vi "D999_Alone.vi"(8 "error in (no error)":errorcluster) -> (0 "error out":errorcluster)   [LabVIEW 2018]
uses:
  RT/PublicSubVI/Ctl/_ctl_RT_D999_Param.ctl
  <resource>/objmgr/ni.var.rc
  <vilib>/Utility/miscctls.llb/LVBoundsTypeDef.ctl
panel:
  in  "D999_list":i32(listbox)=-1
  in  "Load":bool
  in  "Save":bool
  in  "Label":string[](array[string])=["", "", "", "", "", "", "", "", "", "", "", ""]
  in  "AI":string[](array[string])=["AI 0", "AI 1", "AI 2", "AI 3", "AI 4", "AI 5", "AI 6", "AI 7", "AI 8", "AI 9", "AI 10", "AI 11"]
  in  "Multiply":dbl[](array[numeric])=[1.0, 1.0, 1.0, 1.0, 1.0, 1.0, 1.0, 1.0, 1.0, 1.0, 1.0, 1.0]
  in  "Add":dbl[](array[numeric])=[0.0, 0.0, 0.0, 0.0, 0.0, 0.0, 0.0, 0.0, 0.0, 0.0, 0.0, 0.0]
  in  "Enable":bool
  in  "AO":string[](array[string])=["AO 0", "AO 1", "AO 2", "AO 3", "AO 4", "AO 5", "AO 6", "AO 7", "AO 8"]
  in  "WriteValue":i16[](array[numeric])=[0, 0, 0, 0, 0, 0, 0, 0, 0] min=-4095 max=4095
  in  "WriteColor":u32[](array[colorbox])=[16777224, 16777224, 16777224, 16777224, 16777224, 16777224, 16777224, 16777224, 16777224]
  in  "Scale":u16=1 min=1
  in  "CEM(AO1)":bool
  in  "DYNODE(AO 0)":bool
  in  "ESPY(AO2)":bool
  in  "LENS(AO 3 : AO 8)":bool
  in  "Description":string="LENS : OFF; ESPY : OFF; DYNODE : OFF; CEN : OFF; "
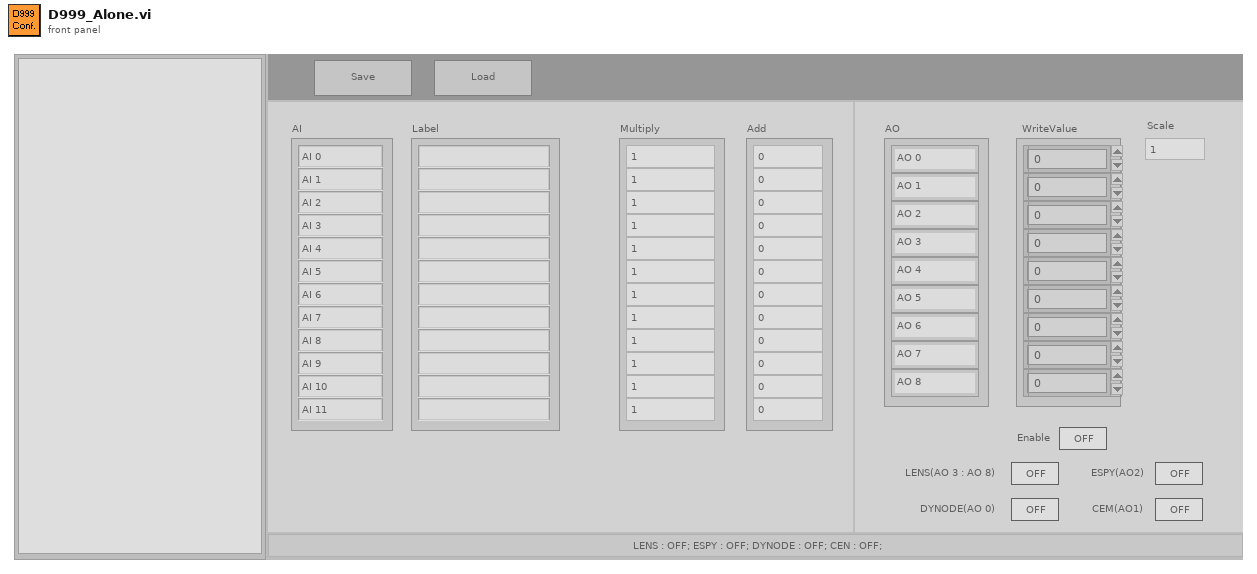
[diagram p1: front panel]
types:
  T1 = cluster{"Enable":refnum<vi>, "Label":refnum<vi>, "Multiply":refnum<vi>, "Add":refnum<vi>, "WriteColor":refnum<vi>, "WriteValue":refnum<vi>, "Description":refnum<vi>, "switch array":refnum<vi>[]}
  T2 = enum8{"Enabled", "Disabled", "Disabled and Grayed Out"}
  T3 = enum32{"Invalid", "Default", "Floating", "Floating/Auto-Hide", "Modal"}
  T4 = typedef "LVBoundsTypeDef.ctl" = cluster{"Width":u32, "Height":u32}
  T5 = cluster{"Label":string, "MultiValue":dbl, "AddValue":dbl}
  T6 = typedef "_ctl_RT_D999_Param.ctl" = cluster{"Enable":bool, "AI":cluster{"Label":string, "MultiValue":dbl, "AddValue":dbl}[], "AO":i16[], "Switch":bool[]}
  T7 = cluster{"Label":string[], "Multiply":dbl[], "Add":dbl[], "WriteValue":i16[], "switch":u32}
  T8 = typedef "eventvkey.ctl" = enum16{"ASCII", "Enter", "Return", "Shift", "Ctrl", "Alt", "Cmd", "Opt", "Caps", "NumLock", "Clear", "Break", "Up", "Down", "Left", "Right", "Insert", "Delete", "Home", "End", "PageUp", "PageDown", "Escape", "Help", "Pause", "ScrollLock", "F1", "F2", "F3", "F4", "F5", "F6", "F7", "F8", "F9", "F10", "F11", "F12", "F13", "F14", "F15", "F16", "F17", "F18", "F19", "F20", "F21", "F22", "F23", "F24", "Play", "VolumeUp", "VolumeDown", "Mute", "Two Byte Char"}
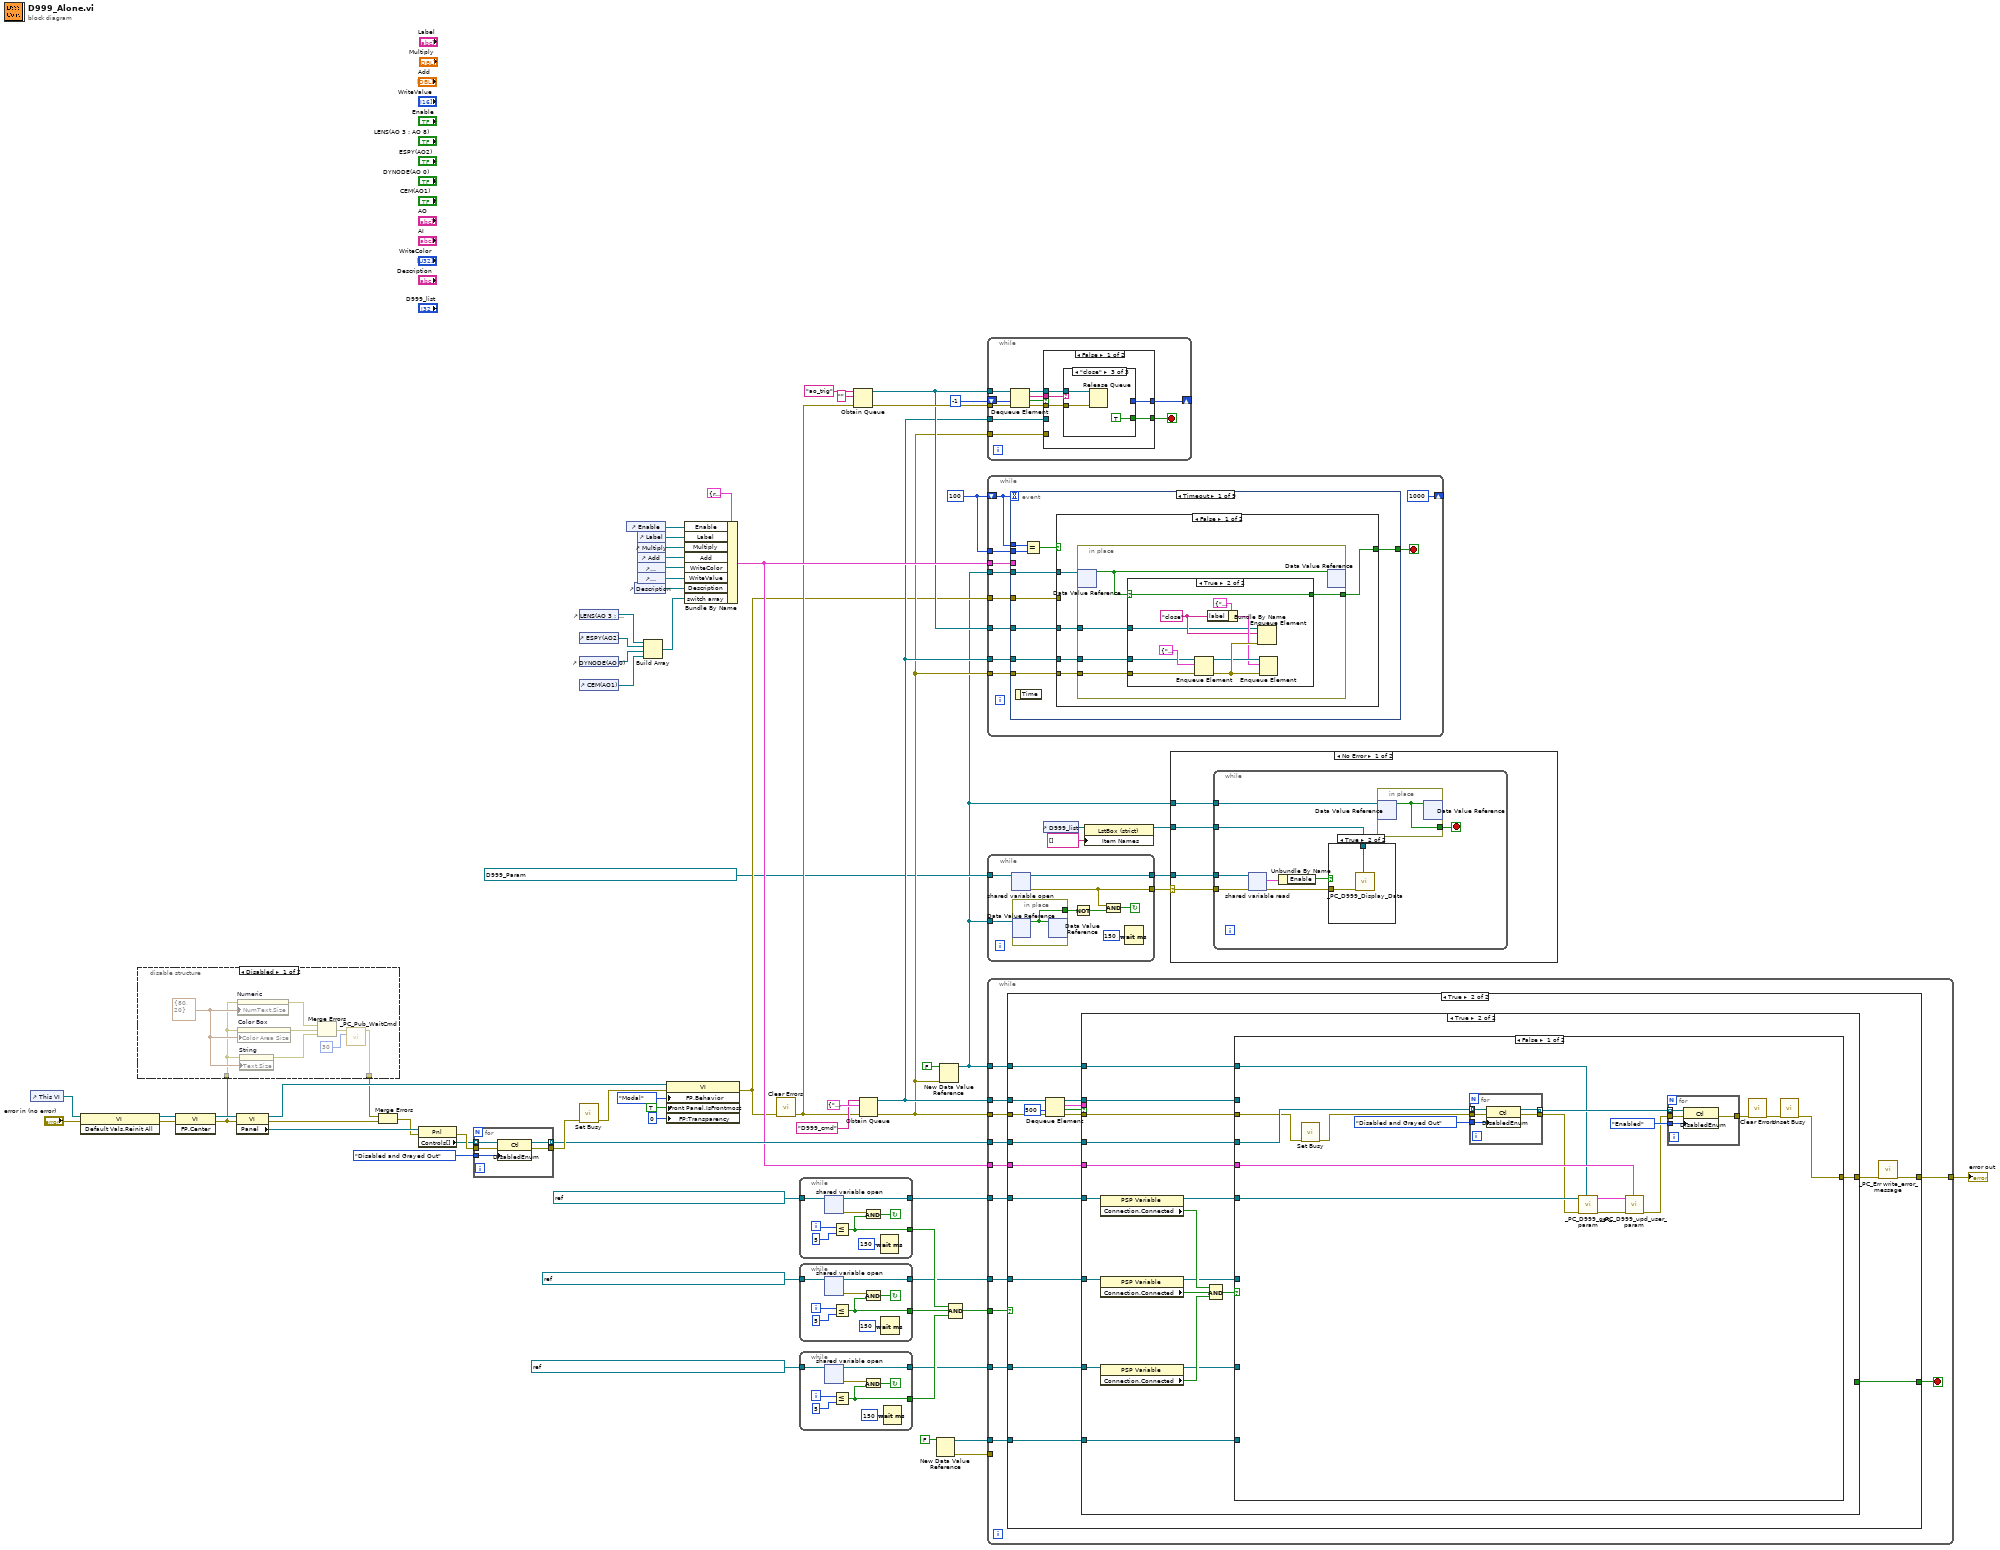
[diagram p0: block diagram]
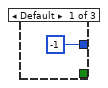
[diagram p5: hidden frame]
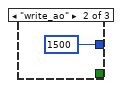
[diagram p6: hidden frame]
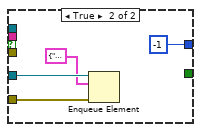
[diagram p7: hidden frame]
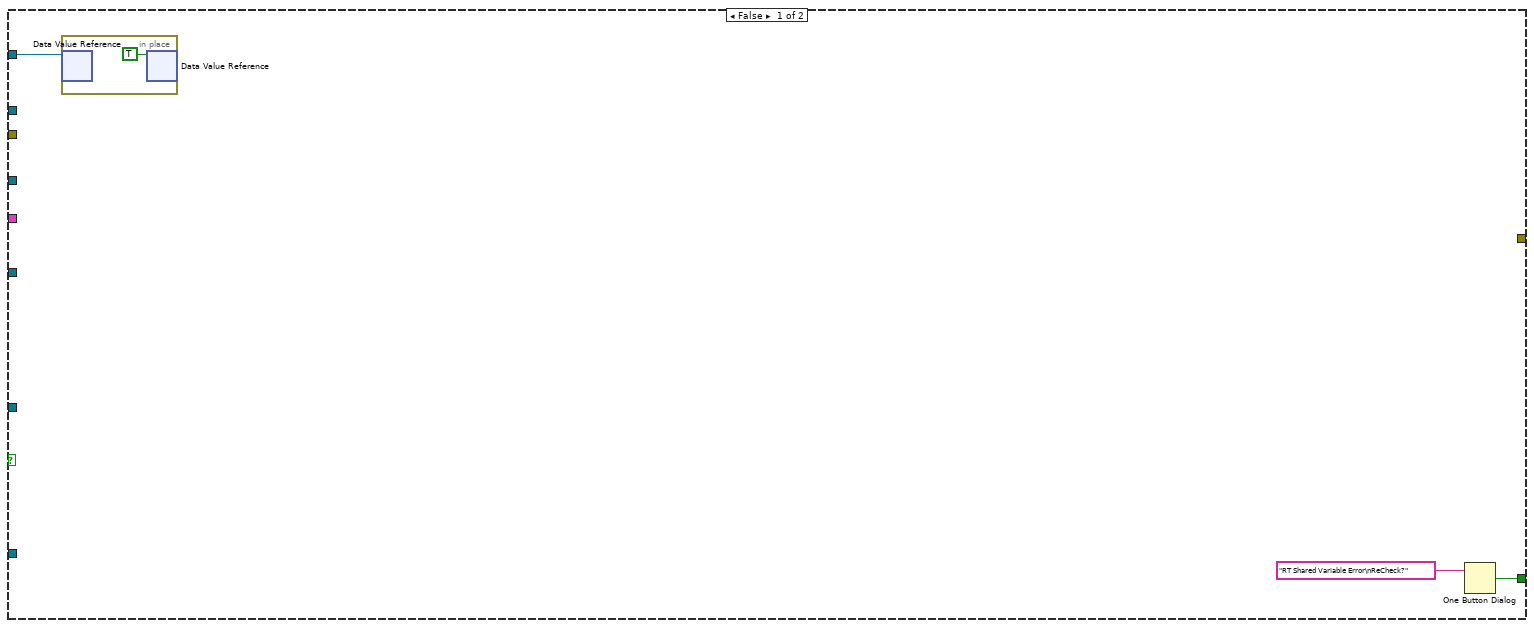
[diagram p8: hidden frame]
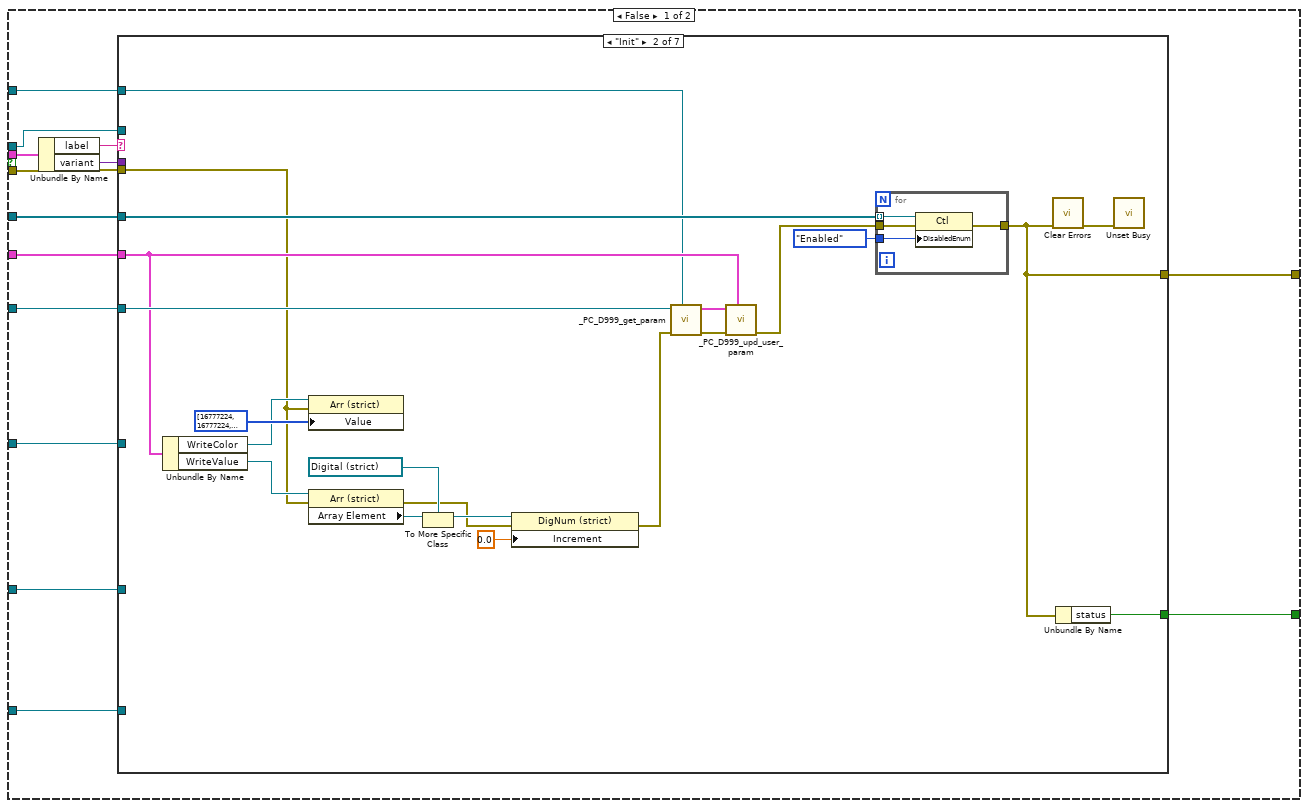
[diagram p9: hidden frame]
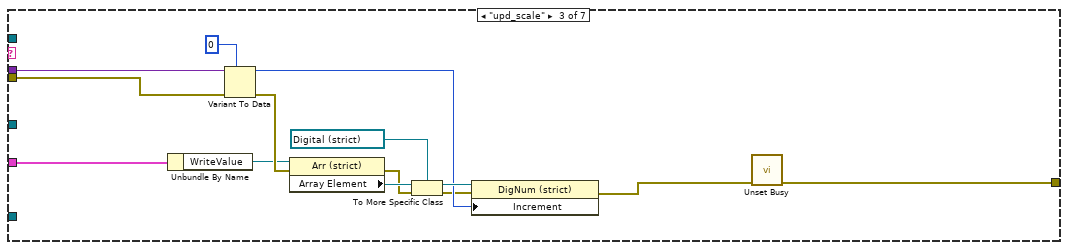
[diagram p11: hidden frame]
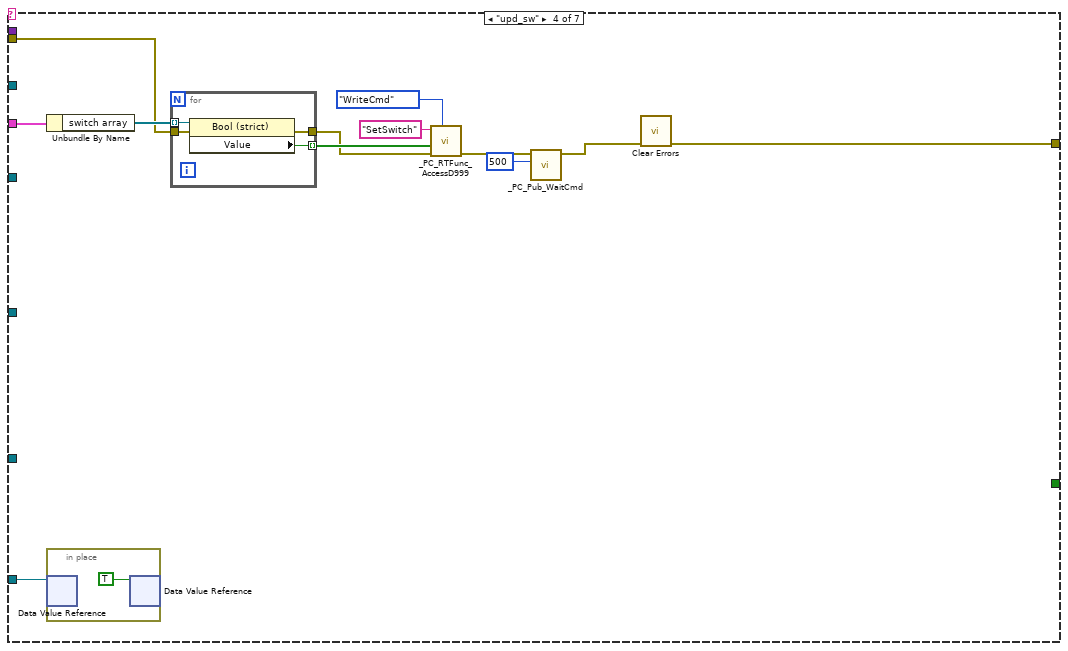
[diagram p12: hidden frame]
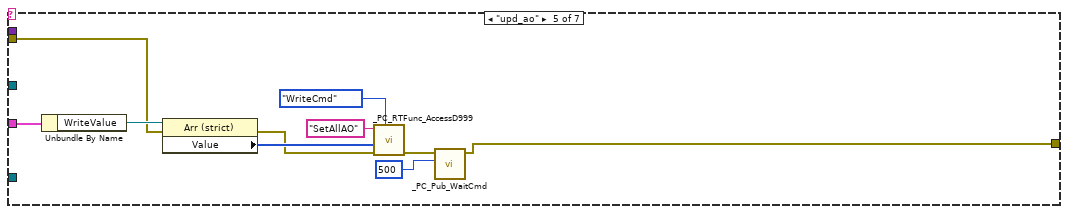
[diagram p13: hidden frame]
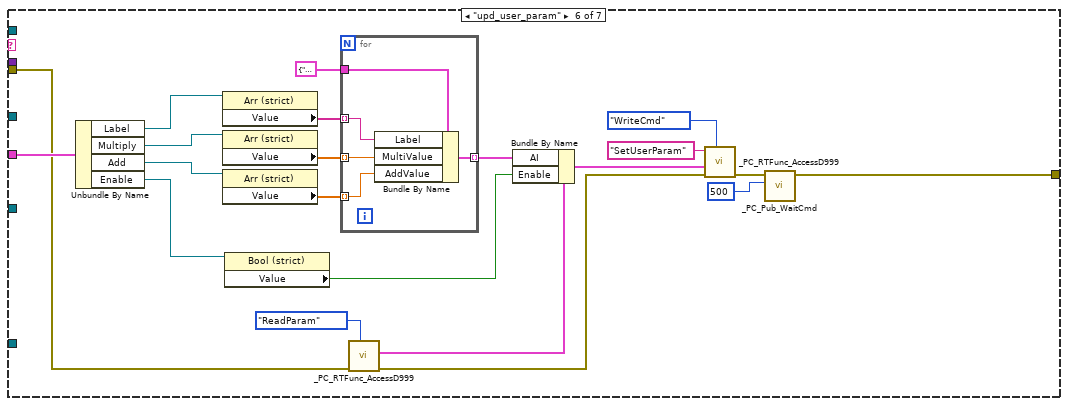
[diagram p14: hidden frame]
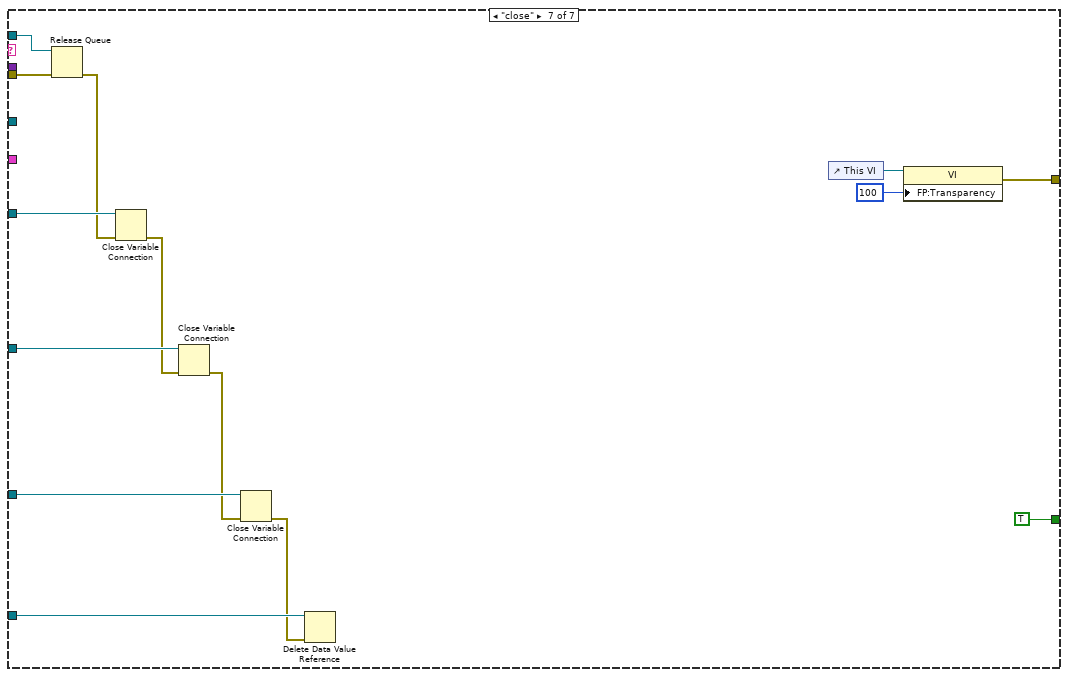
[diagram p15: hidden frame]
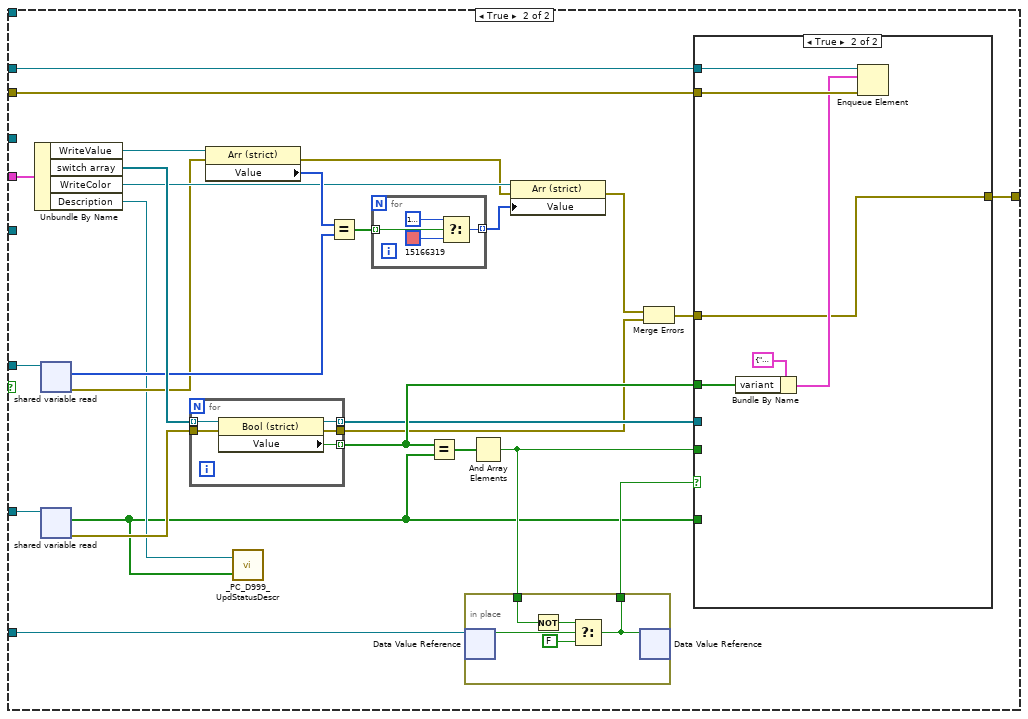
[diagram p16: hidden frame]
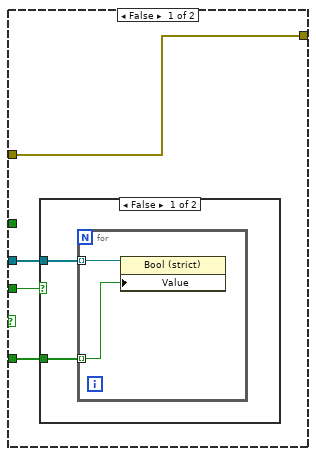
[diagram p17: hidden frame]
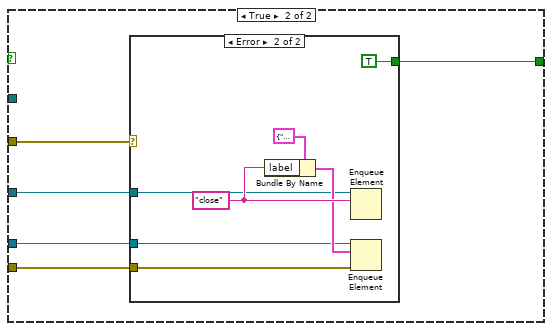
[diagram p20: hidden frame]
diagram:
  w4 = 100
  n1 = control-ref of="This VI"() -> (w65:refnum<vi>)
  n2 = invoke class="VI" method="Default Vals.Reinit All"(reference=w65, error in="error in (no error)") -> (reference out=w66:refnum<vi>, error out=w63:errorcluster)  [unwired: 1 in, 1 out]
  n3 = invoke class="VI" method="FP.Center"(reference=w66, error in=w63) -> (reference out=w58:refnum<vi>, error out=w15:errorcluster)  [unwired: 1 in, 1 out]
  n4 = disable-structure shown="Disabled" {
    disable-tunnel: w15 -> [w70 w77]
    disable-tunnel: [w69 w77] -> w12
    frame Disabled {
      w76 = T4 {"Width"=80, "Height"=20} ("Numeric Text.Size")
      n5 = property on="Numeric" class="DigNum (strict)"(error in=w70, "NumText.Size"=w76) -> (error out=w75:errorcluster)  [unwired: 1 in, 1 out]
      n6 = property on="Color Box" class="ColBox"(error in=w70, "Color Area Size"=w76) -> (error out=w74:errorcluster)  [unwired: 1 in, 1 out]
      n7 = property on="String" class="Str"(error in=w70, "Text.Size"=w76) -> (error out=w73:errorcluster)  [unwired: 1 in, 1 out]
      n8 = Merge Errors(w75, w74, w73) -> (w71:errorcluster)
      n9 = call "_PC_Pub_WaitCmd.vi"("milliseconds to wait"=u32 30, "error in (no error)"=w71) -> ("error out"=w69:errorcluster)  [unwired: 9 in]
    }
    frame Enabled {
    }
  }
  n10 = property class="VI"(reference=w58, error in=w15) -> (reference out=w57:refnum<vi>, error out=w13:errorcluster, "Panel"=w64:refnum<vi>)
  n11 = Merge Errors(w12, w13) -> (w11:errorcluster)
  n12 = property class="Pnl"(reference=w64, error in=w11) -> (error out=w61:errorcluster, "Controls[]"=w60:refnum<vi>[])  [unwired: 1 out]
  n13 = for {
    tunnel: w60 -> [w82] mode=indexing
    tunnel: T2."Disabled and Grayed Out" ("Disabled") -> [w81]
    tunnel: [w80] -> w29 mode=indexing
    tunnel: [w79] -> w56
    tunnel: w61 -> [w78]
    n14 = property class="Ctl"(reference=w82, error in=w78, "DisabledEnum"=w81) -> (reference out=w80:refnum<vi>, error out=w79:errorcluster)
  }
  n15 = control-ref of="LENS(AO 3 : AO 8)"() -> (w40:refnum<vi>)
  n16 = control-ref of="ESPY(AO2)"() -> (w41:refnum<vi>)
  n17 = control-ref of="DYNODE(AO 0)"() -> (w42:refnum<vi>)
  n18 = control-ref of="CEM(AO1)"() -> (w43:refnum<vi>)
  n19 = call <vilib>:"Set Busy.vi"("error in (no error)"=w56) -> ("error out"=w14:errorcluster)  [unwired: 9 in, 1 out]
  n20 = control-ref of="Enable"() -> (w38:refnum<vi>)
  n21 = control-ref of="Description"() -> (w32:refnum<vi>)
  n22 = control-ref of="Label"() -> (w37:refnum<vi>)
  n23 = control-ref of="Multiply"() -> (w36:refnum<vi>)
  n24 = control-ref of="Add"() -> (w35:refnum<vi>)
  n25 = control-ref of="WriteColor"() -> (w34:refnum<vi>)
  n26 = control-ref of="WriteValue"() -> (w33:refnum<vi>)
  n27 = Build Array(w40, w41, w42, w43) -> (w31:refnum<vi>[])
  n28 = property class="VI"(reference=w57, error in=w14, "FP.Behavior"=T3."Modal" ("Front Panel Window:Behavior"), "Front Panel.IsFrontmost"=TRUE ("Front Panel Window:Is Frontmost"), "FP:Transparency"=u8 0 ("Front Panel Window:Transparency")) -> (error out=w10:errorcluster)  [unwired: 1 out]
  n29 = Bundle By Name(cluster=T1 {"Enable"=refnum, "Label"=refnum, "Multiply"=refnum, "Add"=refnum, "WriteColor"=refnum, "WriteValue"=refnum, "Description"=refnum, "switch array"=[]}, "Enable"=w38, "Label"=w37, "Multiply"=w36, "Add"=w35, "WriteColor"=w34, "WriteValue"=w33, "Description"=w32, "switch array"=w31) -> (w26:T1)
  n30 = call <vilib>:"Clear Errors.vi"("error in (no error)"=w10) -> ("error out"=w23:errorcluster)  [unwired: 5 in, 1 out]
  n31 = while {
    tunnel: [w84] -> w51
    tunnel: refnum<k21> "ni.var.psp://NI-sbRIO/_RT_CtrlLoop_D999_Variables/D999_Exist" ("shared variable refnum in") -> [w90]
    tunnel: [w89] -> w52
    i -> [w87]
    stop <- w85 continue-if-true
    n32 = shared-variable-open(w90) -> (w89:refnum<k21>, w86:errorcluster)  [unwired: 1 in]
    n33 = Less Or Equal?(x=w87, y=5) -> (x <= y?=w84:bool)
    n34 = And(x=w86, y=w84) -> (x .and. y?=w85:bool)
    n35 = Wait (ms)(milliseconds to wait=u32 150) -> ()  [unwired: 1 out]
  }
  n36 = while {
    tunnel: [w92] -> w50
    tunnel: refnum<k21> "ni.var.psp://NI-sbRIO/_RT_CtrlLoop_D999_Variables/D999_AO_Res" ("shared variable refnum in") -> [w98]
    tunnel: [w97] -> w45
    i -> [w95]
    stop <- w93 continue-if-true
    n37 = shared-variable-open(w98) -> (w97:refnum<k21>, w94:errorcluster)  [unwired: 1 in]
    n38 = Less Or Equal?(x=w95, y=5) -> (x <= y?=w92:bool)
    n39 = And(x=w94, y=w92) -> (x .and. y?=w93:bool)
    n40 = Wait (ms)(milliseconds to wait=u32 150) -> ()  [unwired: 1 out]
  }
  n41 = while {
    tunnel: [w100] -> w49
    tunnel: refnum<k21> "ni.var.psp://NI-sbRIO/_RT_CtrlLoop_D999_Variables/D999_Switch_Res" ("shared variable refnum in") -> [w106]
    tunnel: [w105] -> w44
    i -> [w103]
    stop <- w101 continue-if-true
    n42 = shared-variable-open(w106) -> (w105:refnum<k21>, w102:errorcluster)  [unwired: 1 in]
    n43 = Less Or Equal?(x=w103, y=5) -> (x <= y?=w100:bool)
    n44 = And(x=w102, y=w100) -> (x .and. y?=w101:bool)
    n45 = Wait (ms)(milliseconds to wait=u32 150) -> ()  [unwired: 1 out]
  }
  n46 = Obtain Queue(name (unnamed)="ao_trig", element data type="", error in (no error)=w23) -> (queue out=w22:refnum<queue>, error out=w24:errorcluster)  [unwired: 2 in, 1 out]
  n47 = Obtain Queue(name (unnamed)="D999_cmd", element data type=cluster{"label":string, "variant":variant} {"label"="", "variant"=variant}, error in (no error)=w23) -> (queue out=w19:refnum<queue>, error out=w16:errorcluster)  [unwired: 2 in, 1 out]
  n48 = New Data Value Reference(data value=FALSE) -> (data value reference=w30:refnum<data-value>, error out=w27:errorcluster)  [unwired: 1 in]
  n49 = New Data Value Reference(data value=FALSE, error in=w16) -> (data value reference=w5:refnum<data-value>)  [unwired: 1 out]
  n50 = Compound Arithmetic op=AND(w51, w50, w49) -> (w48:bool)
  n51 = while {
    tunnel: w22 -> [w117]
    tunnel: w24 -> [w115]
    shift-right: [w110] -> _
    shift-left: -1 ("timeout in ms (-1)") -> [w116]
    tunnel: w19 -> [w108]
    tunnel: w16 -> [w107]
    stop <- w109 stop-if-true
    n52 = Dequeue Element(queue=w117, timeout in ms (-1)=w116, error in (no error)=w115) -> (queue out=w111:refnum<queue>, element=w113:string, timed out?=w114:bool, error out=w112:errorcluster)
    n53 = case shown="False" w114 {
      tunnel: w113 -> [w122 _]
      tunnel: w112 -> [w121 _]
      tunnel: w111 -> [w118 _]
      tunnel: [w120 -1] -> w110
      tunnel: [w119 _] -> w109
      tunnel: w108 -> [_ w130]
      tunnel: w107 -> [_ w129]
      frame False {
        n54 = case shown="\"close\"" w122 {
          tunnel: w121 -> [_ _ w125]
          tunnel: [-1 1500 _] -> w120
          tunnel: [_ _ TRUE] -> w119
          tunnel: w118 -> [_ _ w126]
          frame Default {
          }
          frame "write_ao" {
          }
          frame "close" {
            n55 = Release Queue(queue=w126, error in (no error)=w125) -> ()  [unwired: 1 in, 3 out]
          }
        }
      }
      frame True {
        n56 = Enqueue Element(queue=w130, element=cluster{"label":string, "variant":variant} {"label"="upd_ao", "variant"=variant}, error in (no error)=w129) -> ()  [unwired: 1 in, 3 out]
      }
    }
  }
  n57 = while {
    tunnel: w19 -> [w143]
    tunnel: w16 -> [w142]
    tunnel: w52 -> [w141]
    tunnel: w48 -> [w139]
    tunnel: w45 -> [w138]
    tunnel: w44 -> [w137]
    tunnel: w26 -> [w136]
    tunnel: w30 -> [w135]
    tunnel: w29 -> [w134]
    tunnel: w27 -> [_]
    tunnel: [w133] -> w18
    tunnel: w5 -> [w132]
    stop <- w140 stop-if-true
    n58 = case shown="True" w139 {
      tunnel: w143 -> [_ w164]
      tunnel: w142 -> [_ w163]
      tunnel: w141 -> [_ w158]
      tunnel: [w145 w150] -> w140
      tunnel: w138 -> [_ w157]
      tunnel: w137 -> [_ w156]
      tunnel: w136 -> [_ w155]
      tunnel: w135 -> [_ w153]
      tunnel: w134 -> [_ w152]
      tunnel: [_ w149] -> w133
      tunnel: w132 -> [w144 w148]
      frame False {
        n59 = in-place {
          n60 = in-place-dvr #1(w144) -> ()  [unwired: 2 out]
          n61 = in-place-dvr #1(TRUE ("data value")) -> ()  [unwired: 2 out]
        }
        n62 = One Button Dialog(message="RT Shared Variable Error\nReCheck?") -> (true=w145:bool)  [unwired: 1 in]
      }
      frame True {
        n63 = Dequeue Element(queue=w164, timeout in ms (-1)=500, error in (no error)=w163) -> (queue out=w154:refnum<queue>, element=w159:cluster{"label":string, "variant":variant}, timed out?=w161:bool, error out=w160:errorcluster)
        n64 = case shown="True" w161 {
          tunnel: w160 -> [w170 w291]
          tunnel: w159 -> [w178 _]
          tunnel: w158 -> [w175 w302]
          tunnel: w157 -> [w174 w301]
          tunnel: w156 -> [w173 w300]
          tunnel: w155 -> [w171 w293]
          tunnel: w154 -> [w166 w292]
          tunnel: w153 -> [w169 w290]
          tunnel: w152 -> [w172 w288]
          tunnel: [w168 w287] -> w151
          tunnel: [w167 _] -> w150
          tunnel: w148 -> [w165 w286]
          frame False {
            n65 = Unbundle By Name(w178) -> ("label"=w177:string, "variant"=w176:variant)
            n66 = case shown="\"Init\"" w177 {
              tunnel: w176 -> [_ _ w213 _ _ _ _]
              tunnel: w175 -> [_ w197 _ _ _ _ w282]
              tunnel: w174 -> [_ _ _ _ _ _ w280]
              tunnel: w173 -> [_ _ _ _ _ _ w278]
              tunnel: w172 -> [_ w200 _ _ _ _ _]
              tunnel: w171 -> [_ w193 w209 w225 w240 w254 _]
              tunnel: w170 -> [w179 w184 w205 w220 w238 w247 w283]
              tunnel: w169 -> [_ _ _ w222 _ _ w279]
              tunnel: [w179 w181 w206 w219 w236 w246 w272] -> w168
              tunnel: [_ w180 _ _ _ _ TRUE] -> w167
              tunnel: w166 -> [_ _ _ _ _ _ w284]
              tunnel: w165 -> [_ w182 _ _ _ _ _]
              frame Default {
              }
              frame "Init" {
                n67 = Unbundle By Name(w193) -> ("WriteColor"=w185:refnum<vi>, "WriteValue"=w187:refnum<vi>)
                n68 = property class="Arr (strict)"(reference=w185, error in=w184, "Value"=u32[] [16777224, 16777224, 16777224, 16777224, 16777224, 16777224, 16777224, 16777224, 16777224]) -> ()  [unwired: 2 out]
                n69 = property class="Arr (strict)"(reference=w187, error in=w184) -> (error out=w188:errorcluster, "Array Element"=w192:refnum<vi>)  [unwired: 1 out]
                n70 = To More Specific Class(target class=refnum<vi> refnum ("Numeric"), reference=w192) -> (specific class reference=w189:refnum<vi>)  [unwired: 1 in, 1 out]
                n71 = property class="DigNum (strict)"(reference=w189, error in=w188, "Increment"=0.0 ("Data Entry Limits:Increment")) -> (error out=w183:errorcluster)  [unwired: 1 out]
                n72 = call "_PC_D999_get_param.vi"("stop cmd"=w182, "error in (no error)"=w183, "D999_exist SV"=w197) -> ("error out"=w198:errorcluster, "D999_Param"=w199:T6)  [unwired: 7 in]
                n73 = call "_PC_D999_upd_user_param.vi"("refnum cluster"=w193, "error in (no error)"=w198, "D999_Param"=w199) -> ("error out"=w196:errorcluster)  [unwired: 8 in]
                n74 = for {
                  tunnel: w200 -> [w204] mode=indexing
                  tunnel: T2."Enabled" ("Disabled") -> [w203]
                  tunnel: [w202] -> w181
                  tunnel: w196 -> [w201]
                  n75 = property class="Ctl"(reference=w204, error in=w201, "DisabledEnum"=w203) -> (error out=w202:errorcluster)  [unwired: 1 out]
                }
                n76 = call <vilib>:"Clear Errors.vi"("error in (no error)"=w181) -> ("error out"=w194:errorcluster)  [unwired: 5 in, 1 out]
                n77 = Unbundle By Name(w181) -> ("status"=w180:bool)
                n78 = call <vilib>:"Unset Busy.vi"("error in (no error)"=w194) -> ()  [unwired: 10 in, 1 out]
              }
              frame "upd_scale" {
                n79 = Unbundle By Name(w209) -> ("WriteValue"=w208:refnum<vi>)
                n80 = Variant To Data(error in=w205, type=u16 0 ("NewVal"), Variant=w213) -> (data=w214:u16, error out=w210:errorcluster)
                n81 = property class="Arr (strict)"(reference=w208, error in=w210) -> (error out=w212:errorcluster, "Array Element"=w217:refnum<vi>)  [unwired: 1 out]
                n82 = To More Specific Class(target class=refnum<vi> refnum ("Numeric"), reference=w217, error in=w212) -> (specific class reference=w216:refnum<vi>, error out=w211:errorcluster)
                n83 = property class="DigNum (strict)"(reference=w216, error in=w211, "Increment"=w214) -> (error out=w207:errorcluster)  [unwired: 1 out]
                n84 = call <vilib>:"Unset Busy.vi"("error in (no error)"=w207) -> ("error out"=w206:errorcluster)  [unwired: 10 in]
              }
              frame "upd_sw" {
                n85 = Unbundle By Name(w225) -> ("switch array"=w224:refnum<vi>[])
                n86 = in-place {
                  n87 = in-place-dvr #2(w222) -> ()  [unwired: 2 out]
                  n88 = in-place-dvr #2(TRUE ("data value")) -> ()  [unwired: 2 out]
                }
                n89 = for {
                  tunnel: w224 -> [w235] mode=indexing
                  tunnel: [w234] -> w229 mode=indexing
                  tunnel: w220 -> [w233]
                  tunnel: [w232] -> w223
                  n90 = property class="Bool (strict)"(reference=w235, error in=w233) -> (error out=w232:errorcluster, "Value"=w234:bool)  [unwired: 1 out]
                }
                n91 = call "_PC_RTFunc_AccessD999.vi"("Function"=enum16{"WriteCmd", "ReadParam", "ReadResponse"}."WriteCmd", "error in (no error)"=w223, "Variant"=w229, "Cmd"="SetSwitch") -> ("error out"=w228:errorcluster)  [unwired: 6 in, 1 out]
                n92 = call "_PC_Pub_WaitCmd.vi"("milliseconds to wait"=u32 500, "error in (no error)"=w228) -> ("error out"=w221:errorcluster)  [unwired: 9 in]
                n93 = call <vilib>:"Clear Errors.vi"("error in (no error)"=w221) -> ("error out"=w219:errorcluster)  [unwired: 5 in, 1 out]
              }
              frame "upd_ao" {
                n94 = Unbundle By Name(w240) -> ("WriteValue"=w239:refnum<vi>)
                n95 = property class="Arr (strict)"(reference=w239, error in=w238) -> (error out=w237:errorcluster, "Value"=w244:i16[])  [unwired: 1 out]
                n96 = call "_PC_RTFunc_AccessD999.vi"("Function"=enum16{"WriteCmd", "ReadParam", "ReadResponse"}."WriteCmd", "error in (no error)"=w237, "Variant"=w244, "Cmd"="SetAllAO") -> ("error out"=w243:errorcluster)  [unwired: 6 in, 1 out]
                n97 = call "_PC_Pub_WaitCmd.vi"("milliseconds to wait"=u32 500, "error in (no error)"=w243) -> ("error out"=w236:errorcluster)  [unwired: 9 in]
              }
              frame "upd_user_param" {
                n98 = Unbundle By Name(w254) -> ("Label"=w253:refnum<vi>, "Multiply"=w252:refnum<vi>, "Add"=w251:refnum<vi>, "Enable"=w250:refnum<vi>)
                n99 = property class="Arr (strict)"(reference=w253) -> ("Value"=w263:string[])  [unwired: 1 in, 2 out]
                n100 = property class="Arr (strict)"(reference=w252) -> ("Value"=w262:dbl[])  [unwired: 1 in, 2 out]
                n101 = property class="Arr (strict)"(reference=w251) -> ("Value"=w261:dbl[])  [unwired: 1 in, 2 out]
                n102 = property class="Bool (strict)"(reference=w250) -> ("Value"=w258:bool)  [unwired: 1 in, 2 out]
                n103 = for {
                  tunnel: T5 {"Label"="", "MultiValue"=0.0, "AddValue"=0.0} ("EC_Param Cluster") -> [w271]
                  tunnel: w263 -> [w270] mode=indexing
                  tunnel: w262 -> [w269] mode=indexing
                  tunnel: w261 -> [w268] mode=indexing
                  tunnel: [w267] -> w260 mode=indexing
                  n104 = Bundle By Name(cluster=w271, "Label"=w270, "MultiValue"=w269, "AddValue"=w268) -> (w267:T5)
                }
                n105 = call "_PC_RTFunc_AccessD999.vi"("Function"=enum16{"WriteCmd", "ReadParam", "ReadResponse"}."ReadParam", "error in (no error)"=w247) -> ("error out"=w256:errorcluster, "D999_Param"=w259:T6)  [unwired: 8 in]
                n106 = Bundle By Name(cluster=w259, "AI"=w260, "Enable"=w258) -> (w257:T6)
                n107 = call "_PC_RTFunc_AccessD999.vi"("Function"=enum16{"WriteCmd", "ReadParam", "ReadResponse"}."WriteCmd", "error in (no error)"=w256, "Variant"=w257, "Cmd"="SetUserParam") -> ("error out"=w249:errorcluster)  [unwired: 6 in, 1 out]
                n108 = call "_PC_Pub_WaitCmd.vi"("milliseconds to wait"=u32 500, "error in (no error)"=w249) -> ("error out"=w246:errorcluster)  [unwired: 9 in]
              }
              frame "close" {
                n109 = Release Queue(queue=w284, error in (no error)=w283) -> (error out=w281:errorcluster)  [unwired: 1 in, 2 out]
                n110 = Close Variable Connection(8:w281, 11:w282) -> (0:w277:errorcluster)
                n111 = Close Variable Connection(8:w277, 11:w280) -> (0:w276:errorcluster)
                n112 = Close Variable Connection(8:w276, 11:w278) -> (0:w275:errorcluster)
                n113 = Delete Data Value Reference(data value reference=w279, error in=w275) -> ()  [unwired: 2 out]
                n114 = control-ref of="This VI"() -> (w274:refnum<vi>)
                n115 = property class="VI"(reference=w274, "FP:Transparency"=u8 100 ("Front Panel Window:Transparency")) -> (error out=w272:errorcluster)  [unwired: 1 in, 1 out]
              }
            }
          }
          frame True {
            n116 = property class="PSP Variable"(reference=w302) -> (reference out=w289:refnum<k21>, "Connection.Connected"=w298:bool)  [unwired: 1 in, 1 out]
            n117 = property class="PSP Variable"(reference=w301) -> (reference out=w295:refnum<k21>, "Connection.Connected"=w299:bool)  [unwired: 1 in, 1 out]
            n118 = property class="PSP Variable"(reference=w300) -> (reference out=w294:refnum<k21>, "Connection.Connected"=w297:bool)  [unwired: 1 in, 1 out]
            n119 = Compound Arithmetic op=AND(w298, w299, w297) -> (w296:bool)
            n120 = case shown="False" w296 {
              tunnel: w295 -> [_ w354]
              tunnel: w294 -> [_ w353]
              tunnel: w293 -> [w315 w352]
              tunnel: w292 -> [_ w337]
              tunnel: w291 -> [w306 w338]
              tunnel: w290 -> [_ w347]
              tunnel: w289 -> [w316 _]
              tunnel: w288 -> [w309 _]
              tunnel: [w304 w330] -> w287
              tunnel: w286 -> [w303 _]
              frame False {
                n121 = call <vilib>:"Set Busy.vi"("error in (no error)"=w306) -> ("error out"=w305:errorcluster)  [unwired: 9 in, 1 out]
                n122 = for {
                  tunnel: w309 -> [w323] mode=indexing
                  tunnel: T2."Disabled and Grayed Out" ("Disabled") -> [w322]
                  tunnel: [w321] -> w307
                  tunnel: w305 -> [w320]
                  tunnel: [w319] -> w308 mode=indexing
                  n123 = property class="Ctl"(reference=w323, error in=w320, "DisabledEnum"=w322) -> (reference out=w319:refnum<vi>, error out=w321:errorcluster)
                }
                n124 = call "_PC_D999_get_param.vi"("stop cmd"=w303, "error in (no error)"=w307, "D999_exist SV"=w316) -> ("error out"=w317:errorcluster, "D999_Param"=w318:T6)  [unwired: 7 in]
                n125 = call "_PC_D999_upd_user_param.vi"("refnum cluster"=w315, "error in (no error)"=w317, "D999_Param"=w318) -> ("error out"=w311:errorcluster)  [unwired: 8 in]
                n126 = for {
                  tunnel: w308 -> [w327] mode=indexing
                  tunnel: T2."Enabled" ("Disabled") -> [w326]
                  tunnel: [w325] -> w312
                  tunnel: w311 -> [w324]
                  n127 = property class="Ctl"(reference=w327, error in=w324, "DisabledEnum"=w326) -> (error out=w325:errorcluster)  [unwired: 1 out]
                }
                n128 = call <vilib>:"Clear Errors.vi"("error in (no error)"=w312) -> ("error out"=w313:errorcluster)  [unwired: 5 in, 1 out]
                n129 = call <vilib>:"Unset Busy.vi"("error in (no error)"=w313) -> ("error out"=w304:errorcluster)  [unwired: 10 in]
              }
              frame True {
                n130 = Unbundle By Name(w352) -> ("WriteValue"=w350:refnum<vi>, "switch array"=w351:refnum<vi>[], "WriteColor"=w340:refnum<vi>, "Description"=w329:refnum<vi>)
                n131 = shared-variable-read(w354) -> (w336:errorcluster, w349:i16[])  [unwired: 1 in, 1 out]
                n132 = shared-variable-read(w353) -> (w334:errorcluster, w328:bool[])  [unwired: 1 in, 1 out]
                n133 = for {
                  tunnel: w351 -> [w382] mode=indexing
                  tunnel: [w381] -> w345 mode=indexing
                  tunnel: [w380] -> w342 mode=indexing
                  tunnel: w334 -> [w379]
                  tunnel: [w378] -> w332
                  n134 = property class="Bool (strict)"(reference=w382, error in=w379) -> (reference out=w380:refnum<vi>, error out=w378:errorcluster, "Value"=w381:bool)
                }
                n135 = property class="Arr (strict)"(reference=w350, error in=w336) -> (error out=w335:errorcluster, "Value"=w344:i16[])  [unwired: 1 out]
                n136 = call "_PC_D999_UpdStatusDescr.vi"("Switch Enable"=w328, "Description"=w329) -> ()  [unwired: 1 in]
                n137 = Equal?(x=w344, y=w349) -> (x = y?=w339:bool[])
                n138 = for {
                  tunnel: w339 -> [w358] mode=indexing
                  tunnel: [w355] -> w341 mode=indexing
                  n139 = Select(t=u32 16777224, s=w358, f=u32 15166319) -> (s? t:f=w355:u32)
                }
                n140 = Equal?(x=w345, y=w328) -> (x = y?=w348:bool[])
                n141 = And Array Elements(Boolean array=w348) -> (logical AND=w343:bool)
                n142 = in-place {
                  in-place-border: w343 -> [w376]
                  in-place-border: [w373] -> w346
                  n143 = in-place-dvr #3(w347) -> (w377:bool)  [unwired: 1 out]
                  n144 = Not(x=w376) -> (.not. x?=w375:bool)
                  n145 = Select(t=w375, s=w377, f=FALSE) -> (s? t:f=w373:bool)
                  n146 = in-place-dvr #3(w373) -> ()  [unwired: 2 out]
                }
                n147 = property class="Arr (strict)"(reference=w340, error in=w335, "Value"=w341) -> (error out=w333:errorcluster)  [unwired: 1 out]
                n148 = Merge Errors(w333, w332) -> (w331:errorcluster)
                n149 = case shown="True" w346 {
                  tunnel: w337 -> [_ w372]
                  tunnel: w338 -> [_ w371]
                  tunnel: w345 -> [_ w369]
                  tunnel: w343 -> [w361 _]
                  tunnel: w342 -> [w362 _]
                  tunnel: w328 -> [w360 _]
                  tunnel: w331 -> [w359 w367]
                  tunnel: [w359 w367] -> w330
                  frame False {
                    n150 = case shown="False" w361 {
                      tunnel: w362 -> [w364 _]
                      tunnel: w360 -> [w363 _]
                      frame False {
                        n151 = for {
                          tunnel: w364 -> [w366] mode=indexing
                          tunnel: w363 -> [w365] mode=indexing
                          n152 = property class="Bool (strict)"(reference=w366, "Value"=w365) -> ()  [unwired: 1 in, 2 out]
                        }
                      }
                      frame True {
                      }
                    }
                  }
                  frame True {
                    n153 = Bundle By Name(cluster=cluster{"label":string, "variant":variant} {"label"="upd_sw", "variant"=variant} ("element"), "variant"=w369) -> (w368:cluster{"label":string, "variant":variant})
                    n154 = Enqueue Element(queue=w372, element=w368, error in (no error)=w371) -> ()  [unwired: 1 in, 3 out]
                  }
                }
              }
            }
          }
        }
        n155 = call "_PC_Err write_error_message.vi"("error in"=w151) -> ("error out"=w149:errorcluster)  [unwired: 10 in]
      }
    }
  }
  "error out" <- w18
  n156 = while {
    tunnel: w26 -> [w392]
    shift-right: [1000] -> _
    shift-left: w4 -> [w384]
    tunnel: w10 -> [w389]
    tunnel: w19 -> [w388]
    tunnel: w16 -> [w387]
    tunnel: w22 -> [w386]
    tunnel: w5 -> [w385]
    tunnel: w4 -> [w383]
    stop <- w391 stop-if-true
    n157 = event shown="[0] Timeout" {
      selector: _ -> [_ _ _ _ _ _ _ _ _]
      dyn-events: _ -> [_ _ _ _ _ _ _ _ _]
      timeout: w384 -> [_ _ _ _ _ _ _ _ _]
      tunnel: [w401 _ _ _ _ _ _ TRUE w516] -> w391
      tunnel: w392 -> [_ w442 w449 _ _ _ _ _ _]
      tunnel: w389 -> [w400 _ _ _ _ _ _ _ _]
      tunnel: w388 -> [w399 _ w445 w465 w468 _ w498 w504 w513]
      tunnel: w387 -> [w398 _ w444 w466 w467 w480 w494 w502 w512]
      tunnel: w386 -> [w397 _ _ _ _ w482 _ w505 w514]
      tunnel: w385 -> [w393 _ _ _ _ _ _ w499 w511]
      tunnel: w384 -> [w396 _ _ _ _ _ _ _ _]
      tunnel: w383 -> [w395 _ _ _ _ _ _ _ _]
      event Timeout {
        n158 = event-data() -> ()  [unwired: 1 in, 1 out]
        n159 = Equal?(x=w396, y=w395) -> (x = y?=w394:bool)
        n160 = case shown="False" w394 {
          tunnel: [w405 w427] -> w401
          tunnel: w400 -> [_ w426]
          tunnel: w399 -> [w404 w425]
          tunnel: w398 -> [w403 w424]
          tunnel: w397 -> [w402 w423]
          tunnel: w393 -> [w406 _]
          frame False {
            n161 = in-place {
              in-place-border: [w410] -> w405
              in-place-border: w404 -> [w409]
              in-place-border: w403 -> [w408]
              in-place-border: w402 -> [w407]
              n162 = in-place-dvr #4(w406) -> (w411:bool)  [unwired: 1 out]
              n163 = case shown="True" w411 {
                selector: w411 -> [w412 w422]
                tunnel: [w412 w422] -> w410
                tunnel: w409 -> [_ w415]
                tunnel: w408 -> [_ w414]
                tunnel: w407 -> [_ w413]
                frame False {
                }
                frame True {
                  w416 = "close" ("element")
                  n164 = Enqueue Element(queue=w415, element=cluster{"label":string, "variant":variant} {"label"="upd_user_param", "variant"=variant}, error in (no error)=w414) -> (queue out=w420:refnum<queue>, error out=w421:errorcluster)  [unwired: 1 in, 1 out]
                  n165 = Bundle By Name(cluster=cluster{"label":string, "variant":variant} {"label"="", "variant"=variant} ("element"), "label"=w416) -> (w419:cluster{"label":string, "variant":variant})
                  n166 = Enqueue Element(queue=w413, element=w416, error in (no error)=w421) -> ()  [unwired: 1 in, 3 out]
                  n167 = Enqueue Element(queue=w420, element=w419, error in (no error)=w421) -> ()  [unwired: 1 in, 3 out]
                }
              }
              n168 = in-place-dvr #4(w411) -> ()  [unwired: 2 out]
            }
          }
          frame True {
            n169 = case shown="Error" w426 {
              tunnel: [_ TRUE ("true")] -> w427
              tunnel: w425 -> [w429 w434]
              tunnel: w424 -> [w428 w433]
              tunnel: w423 -> [_ w435]
              frame No Error {
                n170 = Bundle By Name(cluster=cluster{"label":string, "variant":variant} {"label"="", "variant"=variant} ("element"), "label"="Init") -> (w430:cluster{"label":string, "variant":variant})
                n171 = Enqueue Element(queue=w429, element=w430, error in (no error)=w428) -> ()  [unwired: 1 in, 3 out]
              }
              frame Error {
                w437 = "close" ("element")
                n172 = Bundle By Name(cluster=cluster{"label":string, "variant":variant} {"label"="", "variant"=variant} ("element"), "label"=w437) -> (w436:cluster{"label":string, "variant":variant})
                n173 = Enqueue Element(queue=w435, element=w437) -> ()  [unwired: 2 in, 3 out]
                n174 = Enqueue Element(queue=w434, element=w436, error in (no error)=w433) -> ()  [unwired: 1 in, 3 out]
              }
            }
          }
        }
      }
      event "Save": Value Change {
        n175 = event-data() -> ()  [unwired: 1 in, 1 out]
        n176 = call "_PC_D999 config_param.vi"("Enum"=enum8{"None", "Write", "Read"}."Write", "Refnum cluster in"=w442) -> ("error out"=w440:errorcluster)  [unwired: 7 in, 2 out]
        n177 = case shown="Error" w440 {
          frame No Error {
          }
          frame Error {
            n178 = One Button Dialog(message="Save Failure") -> ()  [unwired: 1 in, 1 out]
          }
        }
      }
      event "Load": Value Change {
        n179 = event-data() -> ()  [unwired: 1 in, 1 out]
        n180 = call "_PC_D999 config_param.vi"("Enum"=enum8{"None", "Write", "Read"}."Read", "Refnum cluster in"=w449) -> ("error out"=w448:errorcluster, "data cluster output"=w446:T7, "Refnum cluster out"=w447:T1)  [unwired: 7 in]
        n181 = case shown="No Error" w448 {
          tunnel: w447 -> [w462 _]
          tunnel: w446 -> [w461 _]
          tunnel: w445 -> [w460 _]
          tunnel: w444 -> [w451 _]
          frame No Error {
            n182 = call "_PC_D999 data_collapse.vi"("error in (no error)"=w451, "data cluster in"=w461, "Refnum cluster in"=w462) -> ("error out"=w452:errorcluster)  [unwired: 7 in, 1 out]
            n183 = Enqueue Element(queue=w460, element=cluster{"label":string, "variant":variant} {"label"="upd_user_param", "variant"=variant}, error in (no error)=w452) -> (queue out=w458:refnum<queue>, error out=w459:errorcluster)  [unwired: 1 in, 1 out]
            n184 = Enqueue Element(queue=w458, element=cluster{"label":string, "variant":variant} {"label"="upd_ao", "variant"=variant}, error in (no error)=w459) -> (queue out=w457:refnum<queue>, error out=w456:errorcluster)  [unwired: 1 in, 1 out]
            n185 = Enqueue Element(queue=w457, element=cluster{"label":string, "variant":variant} {"label"="upd_sw", "variant"=variant}, error in (no error)=w456) -> ()  [unwired: 1 in, 3 out]
          }
          frame Error {
            n186 = One Button Dialog(message="Load Failure") -> ()  [unwired: 1 in, 1 out]
          }
        }
      }
      event "LENS(AO 3 : AO 8)", "ESPY(AO2)", "DYNODE(AO 0)", "CEM(AO1)": Value Change {
        n187 = event-data() -> ()  [unwired: 1 in, 1 out]
        n188 = Enqueue Element(queue=w465, element=cluster{"label":string, "variant":variant} {"label"="upd_sw", "variant"=variant}, error in (no error)=w466) -> ()  [unwired: 1 in, 3 out]
      }
      event "Enable": Value Change {
        n189 = event-data() -> ()  [unwired: 1 in, 6 out]
        n190 = Enqueue Element(queue=w468, element=cluster{"label":string, "variant":variant} {"label"="upd_user_param", "variant"=variant}, error in (no error)=w467) -> ()  [unwired: 1 in, 3 out]
      }
      event "WriteValue": Value Change {
        n191 = event-data() -> ("CtlRef"=w479:refnum<vi>, "OldVal"=w478:i16[], "NewVal"=w471:i16[])  [unwired: 1 in]
        n192 = Not Equal?(x=w478, y=w471) -> (x != y?=w477:bool[])
        n193 = Enqueue Element(queue=w482, element="write_ao" ("label"), error in (no error)=w480) -> ()  [unwired: 1 in, 3 out]
        n194 = Search 1D Array(1D array=w477, element=TRUE) -> (index of element=w470:i32)  [unwired: 1 in]
        n195 = Less?(x=w470, y=3) -> (x < y?=w473:bool)
        n196 = Greater Or Equal To 0?(x=w470) -> (x >= 0?=w474:bool)
        n197 = And(x=w474, y=w473) -> (x .and. y?=w472:bool)
        n198 = case shown="True" w472 {
          tunnel: w479 -> [_ w487]
          tunnel: w471 -> [_ w486]
          tunnel: w470 -> [_ w485]
          frame False {
          }
          frame True {
            n199 = Index Array(array=w486, index=w485) -> (element=w484:i16)
            n200 = Less Than 0?(x=w484) -> (x < 0?=w483:bool)
            n201 = case shown="True" w483 {
              tunnel: w487 -> [_ w492]
              tunnel: w486 -> [_ w489]
              tunnel: w485 -> [_ w488]
              frame False {
              }
              frame True {
                n202 = Replace Array Subset(array=w489, new element=i16 0 ("new element/subarray"), index=w488) -> (w490:i16[])
                n203 = property class="Arr (strict)"(reference=w492, "Value"=w490) -> ()  [unwired: 1 in, 2 out]
              }
            }
          }
        }
      }
      event "Scale": Value Change {
        n204 = event-data() -> ("NewVal"=w496:u16)  [unwired: 1 in]
        n205 = call <vilib>:"Set Busy.vi"("error in (no error)"=w494) -> ("error out"=w493:errorcluster)  [unwired: 9 in, 1 out]
        n206 = Bundle By Name(cluster=cluster{"label":string, "variant":variant} {"label"="upd_scale", "variant"=variant}, "variant"=w496) -> (w495:cluster{"label":string, "variant":variant})
        n207 = Enqueue Element(queue=w498, element=w495, error in (no error)=w493) -> ()  [unwired: 1 in, 3 out]
      }
      event Panel Close {
        w507 = "close" ("element")
        n208 = event-data() -> ()  [unwired: 1 in, 1 out]
        n209 = in-place {
          n210 = in-place-dvr #5(w499) -> ()  [unwired: 2 out]
          n211 = in-place-dvr #5(TRUE ("data value")) -> ()  [unwired: 2 out]
        }
        n212 = Enqueue Element(queue=w504, element=cluster{"label":string, "variant":variant} {"label"="upd_user_param", "variant"=variant}, error in (no error)=w502) -> (queue out=w503:refnum<queue>, error out=w500:errorcluster)  [unwired: 1 in, 1 out]
        n213 = Bundle By Name(cluster=cluster{"label":string, "variant":variant} {"label"="", "variant"=variant} ("element"), "label"=w507) -> (w506:cluster{"label":string, "variant":variant})
        n214 = Enqueue Element(queue=w505, element=w507, error in (no error)=w500) -> ()  [unwired: 1 in, 3 out]
        n215 = Enqueue Element(queue=w503, element=w506, error in (no error)=w500) -> ()  [unwired: 1 in, 3 out]
      }
      event Key Down? {
        n216 = event-data() -> ("VKey"=w515:T8)  [unwired: 1 in]
        n217 = case shown="\"Escape\"" w515 {
          tunnel: [_ TRUE] -> w516
          tunnel: w514 -> [_ w520]
          tunnel: w513 -> [_ w519]
          tunnel: w512 -> [_ w518]
          tunnel: w511 -> [_ w517]
          frame "ASCII", Default {
          }
          frame "Escape" {
            w525 = "close" ("element")
            n218 = in-place {
              n219 = in-place-dvr #6(w517) -> ()  [unwired: 2 out]
              n220 = in-place-dvr #6(TRUE ("data value")) -> ()  [unwired: 2 out]
            }
            n221 = Enqueue Element(queue=w519, element=cluster{"label":string, "variant":variant} {"label"="upd_user_param", "variant"=variant}, error in (no error)=w518) -> (queue out=w523:refnum<queue>, error out=w521:errorcluster)  [unwired: 1 in, 1 out]
            n222 = Bundle By Name(cluster=cluster{"label":string, "variant":variant} {"label"="", "variant"=variant} ("element"), "label"=w525) -> (w524:cluster{"label":string, "variant":variant})
            n223 = Enqueue Element(queue=w520, element=w525, error in (no error)=w521) -> ()  [unwired: 1 in, 3 out]
            n224 = Enqueue Element(queue=w523, element=w524, error in (no error)=w521) -> ()  [unwired: 1 in, 3 out]
          }
        }
        n225 = event-data("Discard?"=w516) -> ()  [unwired: 1 in, 1 out]
      }
    }
  }
  n226 = while {
    tunnel: refnum<k21> "ni.var.psp://NI-sbRIO/_RT_CtrlLoop_D999_Variables/D999_UserParam" ("shared variable refnum in") -> [w536]
    tunnel: w5 -> [w534]
    tunnel: [w530] -> w7
    tunnel: [w529] -> w6
    stop <- w531 continue-if-true
    n227 = shared-variable-open(w536) -> (w530:refnum<k21>, w529:errorcluster)  [unwired: 1 in]
    n228 = in-place {
      in-place-border: [w537] -> w533
      n229 = in-place-dvr #7(w534) -> (w537:bool)  [unwired: 1 out]
      n230 = in-place-dvr #7(w537) -> ()  [unwired: 2 out]
    }
    n231 = Not(x=w533) -> (.not. x?=w532:bool)
    n232 = And(x=w529, y=w532) -> (x .and. y?=w531:bool)
    n233 = Wait (ms)(milliseconds to wait=u32 150) -> ()  [unwired: 1 out]
  }
  n234 = control-ref of="D999_list"() -> (w3:refnum<vi>)
  n235 = property class="LstBox (strict)"(reference=w3, "Item Names"=string[] []) -> (reference out=w2:refnum<vi>)  [unwired: 1 in, 1 out]
  n236 = case shown="No Error" w6 {
    selector: w6 -> [w540 _]
    tunnel: w7 -> [w541 _]
    tunnel: w2 -> [w539 _]
    tunnel: w5 -> [w538 _]
    frame No Error {
      n237 = while {
        tunnel: w541 -> [w549]
        tunnel: w540 -> [w548]
        tunnel: w539 -> [w546]
        tunnel: w538 -> [w543]
        stop <- w542 stop-if-true
        n238 = shared-variable-read(w549, w548) -> (w547:errorcluster, w545:T6)  [unwired: 1 out]
        n239 = Unbundle By Name(w545) -> ("Enable"=w544:bool)
        n240 = case shown="True" w544 {
          tunnel: w547 -> [_ w552]
          tunnel: w546 -> [_ w551]
          frame False {
          }
          frame True {
            n241 = call "_PC_D999_Display_Data.vi"("Listbox"=w551, "error in"=w552) -> ()  [unwired: 9 in, 1 out]
          }
        }
        n242 = in-place {
          in-place-border: [w550] -> w542
          n243 = in-place-dvr #8(w543) -> (w550:bool)  [unwired: 1 out]
          n244 = in-place-dvr #8(w550) -> ()  [unwired: 2 out]
        }
      }
    }
    frame Error {
    }
  }
